vi "Resolve Variable.vi"(8 "error in (no error)":errorcluster, 9 "Variable":string, 10 "Namespace":string, 11 "BasicTemplater in":refnum<class "BasicTemplater.lvclass">) -> (0 "error out":errorcluster, 2 "Value":string, 3 "BasicTemplater out":refnum<class "BasicTemplater.lvclass">)   [LabVIEW 2020, in "HTTP Server.lvlib" / "BasicTemplater.lvclass"]
uses:
  BasicTemplater.lvclass
  BasicTemplater.lvclass/BasicTemplater.ctl
  TemplateVariableResolver/TemplateVariableResolver.lvclass
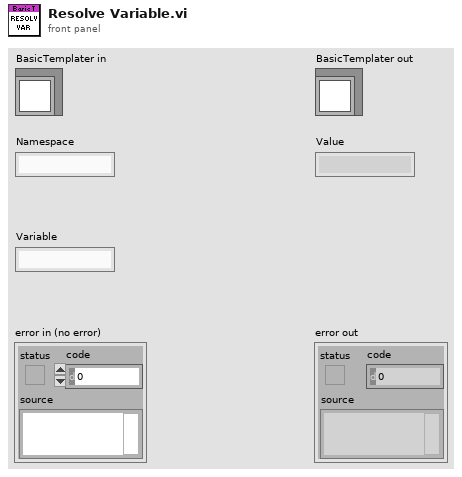
[diagram p1: front panel]
types:
  T1 = map{string, refnum<class "TemplateVariableResolver.lvclass">}
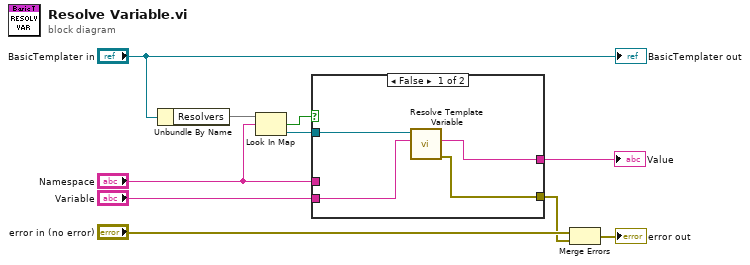
[diagram p0: block diagram]
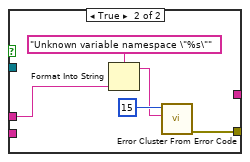
[diagram p2: hidden frame]
diagram:
  n1 = Unbundle By Name("BasicTemplater in") -> ("Resolvers"=w9:T1)
  n2 = Look In Map(map=w9, key="Namespace") -> (key not found?=w3:bool, value=w2:refnum<class "TemplateVariableResolver.lvclass">)  [unwired: 1 in]
  n3 = case shown="False" w3 {
    tunnel: w2 -> [w13 _]
    tunnel: "Namespace" -> [_ w16]
    tunnel: "Variable" -> [w12 _]
    tunnel: [w11 _] -> w6
    tunnel: [w14 w19] -> w4
    frame False {
      n4 = call-dynamic "Resolve Template Variable.vi"("Variable Name"=w12, "TemplateVariableResolver in"=w13) -> ("error out"=w14:errorcluster, "Value"=w11:string)  [unwired: 8 in]
    }
    frame True {
      n5 = Format Into String(format string="Unknown variable namespace \"%s\"", w16) -> (resulting string=w15:string)  [unwired: 2 in, 1 out]
      n6 = call <vilib>:"Error Cluster From Error Code.vi"("error message (\"\")"=w15, "error code (0)"=15) -> ("error out"=w19:errorcluster)  [unwired: 7 in]
    }
  }
  "Value" <- w6
  n7 = Merge Errors("error in (no error)", w4) -> (→"error out":errorcluster)
  "BasicTemplater out" <- "BasicTemplater in"
